vi "Acquire Blob Lease.vi"(6 "Lease duration in seconds (-1: infinite)":i32=-1, 8 "error in (no error)":errorcluster, 9 "Blob":string, 10 "Container":string, 11 "Azure Session in":refnum<class "Session.lvclass">) -> (0 "error out":errorcluster, 2 "Lease ID":string, 3 "Azure Session out":refnum<class "Session.lvclass">)   [LabVIEW 2015, in "NI_Azure_Blob.lvlib"]
doc: "Request a new lease for a blob."
uses:
  NI_Azure_Blob.lvlib
  Core/Session/Session.lvclass
  Core/Name Value Pair.ctl
  Lease Action.ctl
  Core/Session/Session.lvclass/Session.ctl
  Core/Session/Write Request Headers.vi
  Core/Session/Write Request Parameters.vi
  Core/Session/Write HTTP Verb.vi
  Core/Session/Write URL Suffix.vi
  Strings Global.vi
  Core/NI_Azure_Core.lvlib
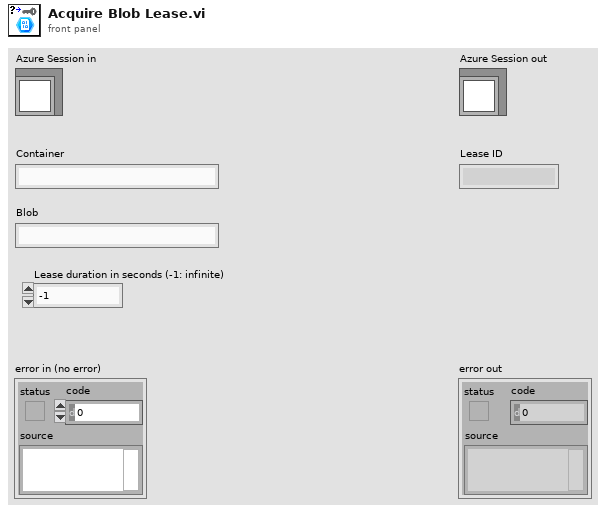
[diagram p1: front panel]
types:
  T1 = typedef "NI_Azure_Blob.lvlib/Lease Action.ctl" = enum16{"acquire", "renew", "change", "release", "break"}
  T2 = typedef "NI_Azure_Core.lvlib/Name Value Pair.ctl" = cluster{"name":string, "value":string}
  T3 = typedef "NI_Azure_Core.lvlib/Response.ctl" = cluster{"Headers":string, "Body":string}
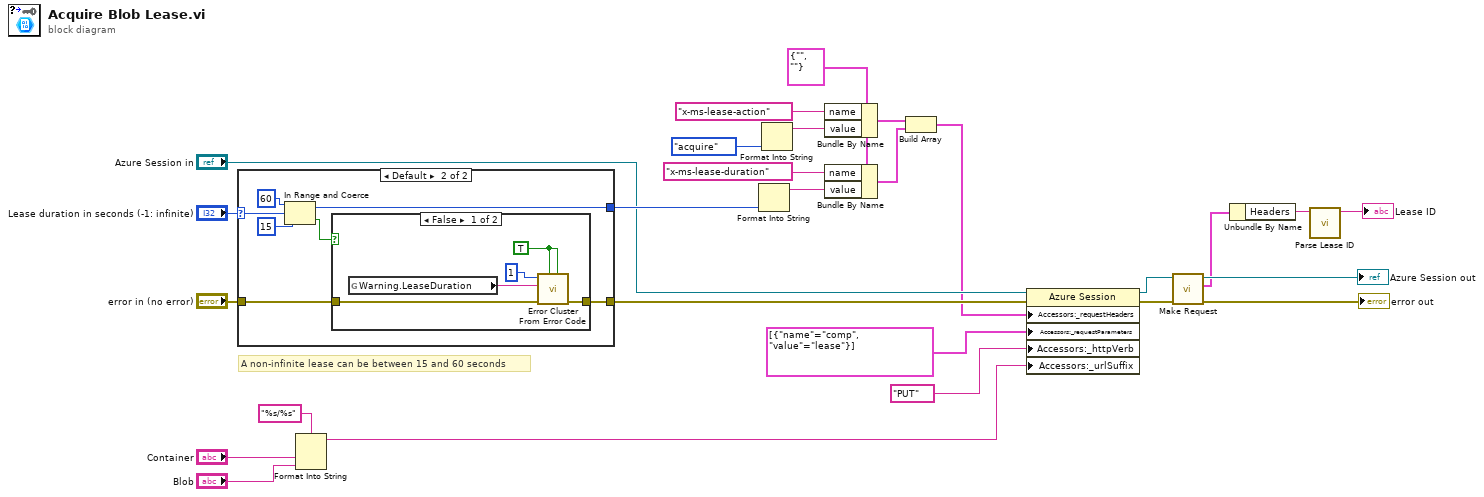
[diagram p0: block diagram]
diagram:
  w16 = T2 {"name"="", "value"=""} ("Cluster")
  # "A non-infinite lease can be between 15 and 60 seconds"
  n1 = case shown="Default" "Lease duration in seconds (-1: infinite)" {
    selector: "Lease duration in seconds (-1: infinite)" -> [w29 w34]
    tunnel: [w29 w33] -> w10
    tunnel: "error in (no error)" -> [w28 w32]
    tunnel: [w28 w31] -> w9
    frame -1 {
    }
    frame Default {
      n2 = In Range and Coerce(upper limit=60, x=w34, lower limit=15) -> (coerced(x)=w33:i32, In Range?=w30:bool)
      n3 = case shown="False" w30 {
        tunnel: w32 -> [w40 w42]
        tunnel: [w39 w42] -> w31
        frame False {
          w41 = TRUE ("show call chain? (False)")
          n4 = global read "Strings Global.vi" "Warning.LeaseDuration"() -> (w37:string)
          n5 = call <vilib>:"Error Cluster From Error Code.vi"("is warning? (False)"=w41, "show call chain? (False)"=w41, "error in (no error)"=w40, "error message (\"\")"=w37, "error code (0)"=1) -> ("error out"=w39:errorcluster)  [unwired: 4 in]
        }
        frame True {
        }
      }
    }
  }
  n6 = Format Into String(format string="%s/%s", "Container", "Blob") -> (resulting string=w1:string)  [unwired: 2 in, 1 out]
  n7 = Format Into String(w10) -> (resulting string=w14:string)  [unwired: 3 in, 1 out]
  n8 = Format Into String(Lease_Action."acquire" ("Lease action")) -> (resulting string=w18:string)  [unwired: 3 in, 1 out]
  n9 = Bundle By Name(cluster=w16, "name"="x-ms-lease-action" ("header"), "value"=w18) -> (w20:T2)
  n10 = Bundle By Name(cluster=w16, "name"="x-ms-lease-duration" ("header"), "value"=w14) -> (w13:T2)
  n11 = Build Array(w20, w13) -> (w4:T2[])
  n12 = property class="Azure Session"(reference="Azure Session in", error in=w9, "Accessors:_requestHeaders"=w4, "Accessors:_requestParameters"=T2[] [{"name"="comp", "value"="lease"}] ("request parameters"), "Accessors:_httpVerb"="PUT" ("HTTP-Verb"), "Accessors:_urlSuffix"=w1) -> (reference out=w5:refnum<class "Session.lvclass">, error out=w7:errorcluster)
  n13 = call "Make Request.vi"("error in (no error)"=w7, "Session in"=w5) -> ("error out"=→"error out":errorcluster, "Response"=w8:T3, "Session out"=→"Azure Session out":refnum<class "Session.lvclass">)  [unwired: 7 in]
  n14 = Unbundle By Name(w8) -> ("Headers"=w12:string)
  n15 = call "Parse Lease ID.vi"("String"=w12) -> ("Lease id"=→"Lease ID":string)  [unwired: 10 in]
